vi "2023 Robot Global Data.vi"() -> ()   [LabVIEW 2020]
doc: "This global VI can contain as many global variables as you need. Place a control on the panel, give it a good name. To read or write to it from a VI, drag the icon to the diagram of that VI. You can also drag from the project. Click on the node to change which global you access. You shouldn't have multiple locations writing to a global or it will cause a race-condition."
uses:
  <vilib>/Rock Robotics/WPI/Camera/WPI_CameraImageSize.ctl
  <vilib>/Rock Robotics/WPI/ThirdParty/Phoenix-LabVIEW/Motor Controller/Controls/CTRE_Phoenix_MotorControl_ControlMode.ctl
panel:
  out "ArmAndWristInitialized":bool
  out "reinitWristPidController":bool
  out "Init Arm Position Settings":bool
  out "reinitArmPidController":bool
  in  "Wrist PID Constants":T1={"P Gain"=0.0, "I Gain"=0.0, "D Gain"=0.0, "F Gain"=0.0, "I Zone"=0.0, "Min Output"=-1.0, "Max Output"=1.0}
  in  "wristSensorPosition":dbl
  in  "wristInitCounter":sgl
  out "Init Wrist Position Settings":bool
  in  "wristMotionRange":dbl=7.0
  in  "wristMaximumPosition":dbl
  in  "wristMinimumPosition":dbl
  in  "wristSetpoint":dbl
  in  "wristMaximumPercentVBusUp":dbl=0.4
  in  "wristMaximumPercentVBusDown":dbl=-0.3
  in  "wristMaximumVelocityUp":dbl=1.0
  in  "wristMaximumVelocityDown":dbl=-1.0
  in  "wristAlpha":dbl
  in  "wristKi":dbl
  in  "wristKd":dbl
  in  "wristKp":dbl=0.005
  in  "armSensorPosition":dbl
  in  "armCounter":i32
  in  "armMaximumPercentVBusUp":dbl=0.4
  in  "armMaximumVelocityUp":dbl=1.0
  in  "joystickDeadband":dbl=0.15
  in  "armMaximumPercentVBusDown":dbl=-0.3
  in  "armMotionRange":dbl=7.0
  in  "armMaximumVelocityDown":dbl=-1.0
  in  "armAlpha":dbl
  in  "Arm PID Constants":T1={"P Gain"=0.0, "I Gain"=0.0, "D Gain"=0.0, "F Gain"=0.0, "I Zone"=0.0, "Min Output"=-1.0, "Max Output"=1.0}
  in  "armMaximumPosition":dbl
  in  "armMinimumPosition":dbl
  in  "armSetpoint":dbl
  in  "armKi":dbl
  in  "armKd":dbl
  in  "armKp":dbl=0.005
  in  "decreaseDriveResponse":dbl=0.6
  in  "driveControl Mode":T2 items=["PercentOutput"=0, "Position"=1, "Velocity"=2, "Current"=3, "Follower"=5, "MotionProfile"=6, "MotionMagic"=7, "MotionProfileArc"=10, "Disabled"=15]
  in  "robotID":string="981-2023"
  in  "imagesize":T3=enum."320x240"
  in  "Enable Vision":bool
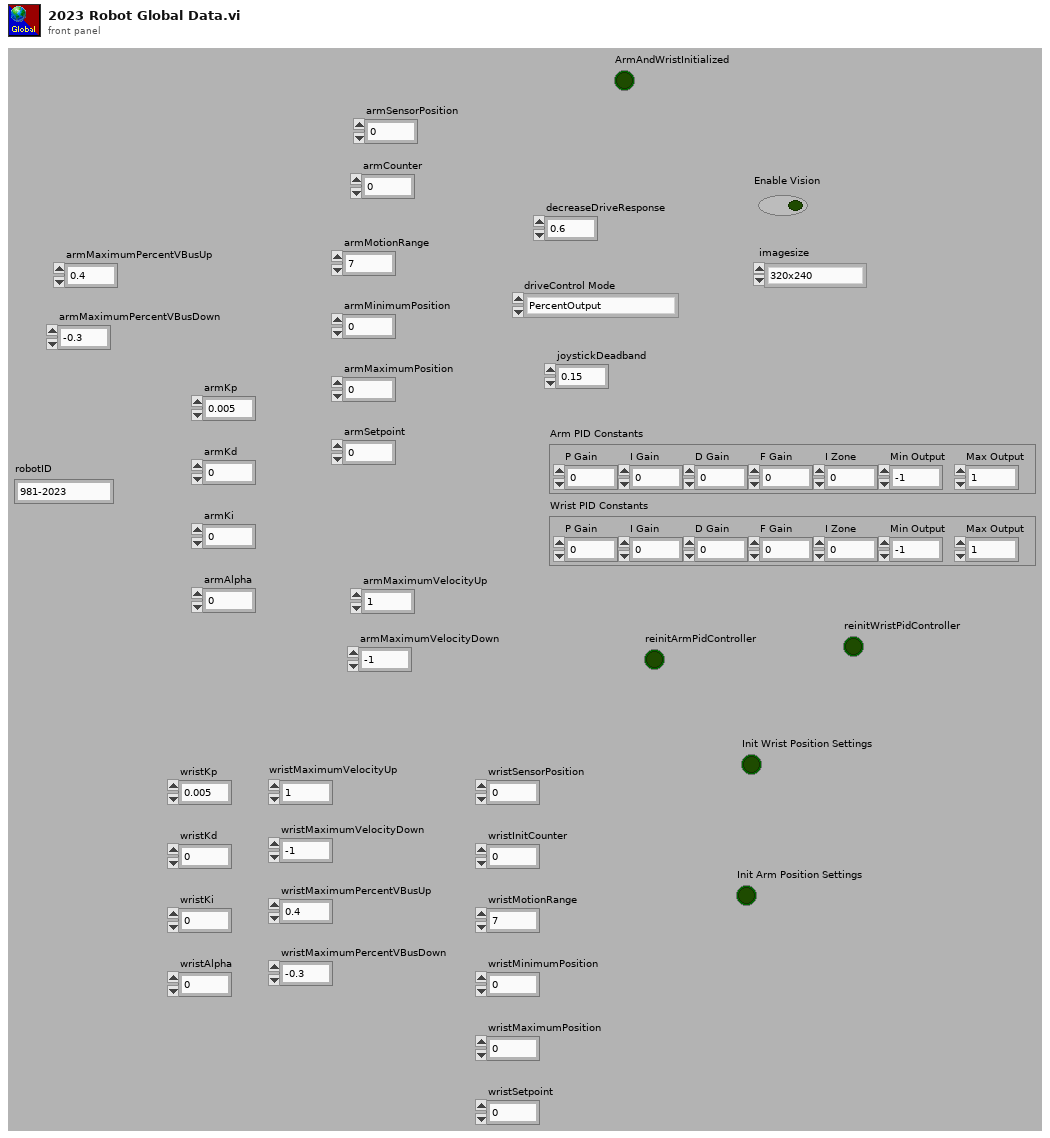
[diagram p1: front panel]
types:
  T1 = cluster{"P Gain":dbl, "I Gain":dbl, "D Gain":dbl, "F Gain":dbl, "I Zone":dbl, "Min Output":dbl, "Max Output":dbl}
  T2 = typedef "CTRE_Phoenix_MotorControl_ControlMode.ctl" = u16
  T3 = typedef "WPI_CameraImageSize.ctl" = enum16{"640x480", "320x240", "160x120", "Custom"}
diagram:
